vi "Read_error.vi"(8 "error in (no error)":errorcluster, 11 "VISA resource in":refnum<visa-resource-name>) -> (0 "error out":errorcluster, 2 "OK":bool, 3 "VISA resource out":refnum<visa-resource-name>)   [LabVIEW 2014, in "B&K Precision 9120 series.lvclass"]
uses:
  B&K Precision 9120 series.lvclass
panel:
  out "system error":string
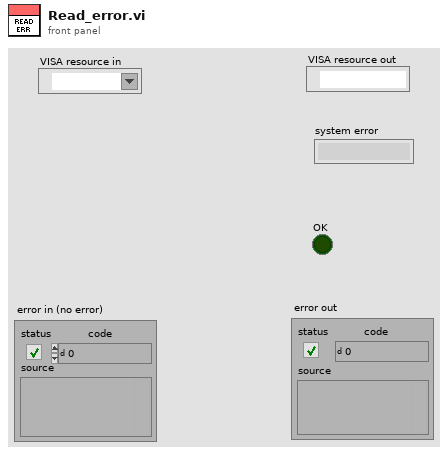
[diagram p1: front panel]
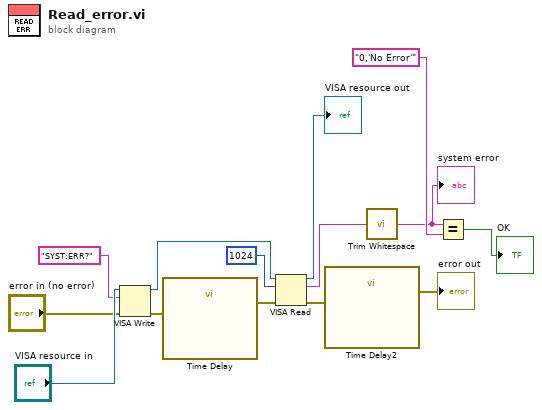
[diagram p0: block diagram]
diagram:
  n1 = VISA Write(VISA resource name="VISA resource in", write buffer="SYST:ERR?", error in (no error)="error in (no error)") -> (VISA resource name out=w11:refnum<visa-resource-name>, error out=w4:errorcluster)  [unwired: 1 out]
  n2 = call "Time Delay"("error in (no error)"=w4) -> ("error out"=w3:errorcluster)  [unwired: 10 in]
  n3 = VISA Read(VISA resource name=w11, byte count=u32 1024, error in (no error)=w3) -> (VISA resource name out=→"VISA resource out":refnum<visa-resource-name>, read buffer=w6:string, error out=w2:errorcluster)  [unwired: 1 out]
  n4 = call "Time Delay2"("error in (no error)"=w2) -> ("error out"=→"error out":errorcluster)  [unwired: 10 in]
  n5 = call <vilib>:"Trim Whitespace.vi"("string"=w6) -> ("trimmed string"=w5:string)  [unwired: 1 in]
  "system error" <- w5
  n6 = Equal?(x=w5, y="0,'No Error'") -> (x = y?=→"OK":bool)
